vi "svc_Get Waveform Subset (Index).vi"(8 "error in (no error)":errorcluster, 9 "length (-1 = all)":i32=-1 min=-1 step=1, 10 "start index (0)":i32 step=1, 11 "waveform in":waveform(dbl)) -> (0 "error out":errorcluster, 1 "actual length":i32, 2 "actual start index":i32, 3 "waveform subset":waveform(dbl), 4 "end reached":bool, 5 "subset timestamp":timestamp)   [LabVIEW 2017]
doc: "Returns a portion of the waveform of the <B>start index</B> and <B>length</B> values. When you wire a waveform to this VI, the waveform automatically resizes to display <B>start index</B> inputs for the waveform."
uses:
  <vilib>/addons/_NISVFA/_Shared subVIs/Common/svc_Coerce Index and Length.vi
  <vilib>/addons/_NISVFA/_Shared subVIs/Common/svc_Conditional Merge Error.vi
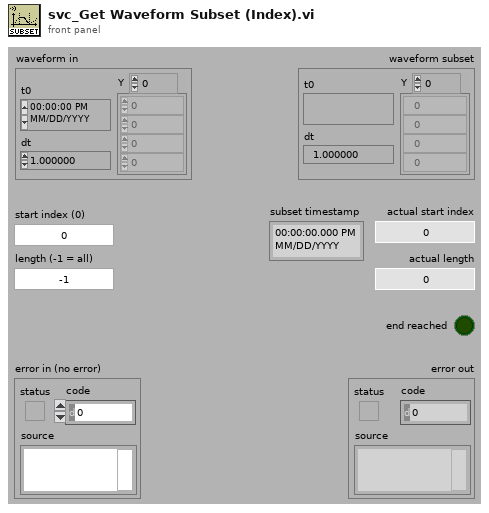
[diagram p1: front panel]
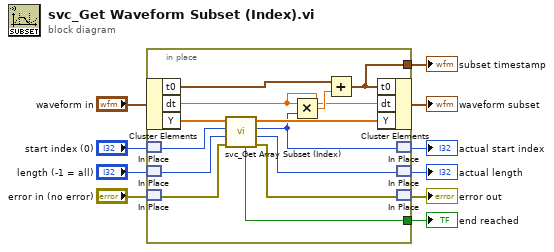
[diagram p0: block diagram]
diagram:
  n1 = in-place {
    in-place-border: [w14] -> w6
    in-place-border: [w11] -> w1
    n2 = in-place-cluster #1("waveform in") -> ("t0"=w22:timestamp, "dt"=w21:dbl, "Y"=w20:dbl[])
    n3 = in-place-match #2("start index (0)") -> (w19:i32)
    n4 = in-place-match #3("length (-1 = all)") -> (w18:i32)
    n5 = in-place-match #4("error in (no error)") -> (w13:errorcluster)
    n6 = call <vilib>:"svc_Get Array Subset (Index).vi"("error in (no error)"=w13, "length (-1 = all)"=w18, "start index (0)"=w19, "Y"=w20) -> ("error out"=w12:errorcluster, "actual length"=w16:i32, "actual start index"=w15:i32, "Y subset"=w17:dbl[], "end reached"=w14:bool)  [unwired: 3 in]
    n7 = Multiply(x=w21, y=w15) -> (x*y=w23:dbl)
    n8 = Add(x=w22, y=w23) -> (x+y=w11:timestamp)
    n9 = in-place-cluster #1("t0"=w11, "dt"=w21, "Y"=w17) -> (→"waveform subset":waveform(dbl))
    n10 = in-place-match #2(w15) -> (→"actual start index":i32)
    n11 = in-place-match #3(w16) -> (→"actual length":i32)
    n12 = in-place-match #4(w12) -> (→"error out":errorcluster)
  }
  "end reached" <- w6
  "subset timestamp" <- w1
